vi "Event Status Enable.vi"(0 "Instrument Handle In":i32, 1 "Status Register":i32 format="%02x", 2 "Frequency Register":i32 format="%02x", 3 "Test Register":i32 format="%04x", 4 "Operation Register":i32 format="%04x", 5 "error in":errorcluster, 6 "Standard Register":i32 format="%02x", 7 "Questionable Register":i32 format="%04x", 8 "Voltage Register":i32 format="%02x", 9 "Calibration Register":i32 format="%02x", 10 "Dig1 Register":i32 caption="Digitizer 1 Register" format="%02x", 11 "Dig2 Register":i32 caption="Digitizer 2 Register" format="%02x") -> (14 "Instrument Handle Out":i32, 19 "error out":errorcluster)   [LabVIEW 8.6, in "ZTScopeM.lvlib"]
doc: "Set all error register event forwarding states."
uses:
  ZTScopeM.lvlib
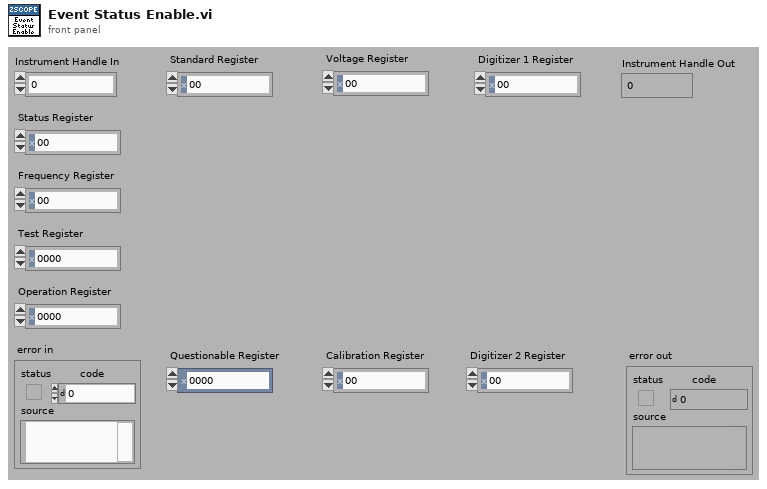
[diagram p1: front panel]
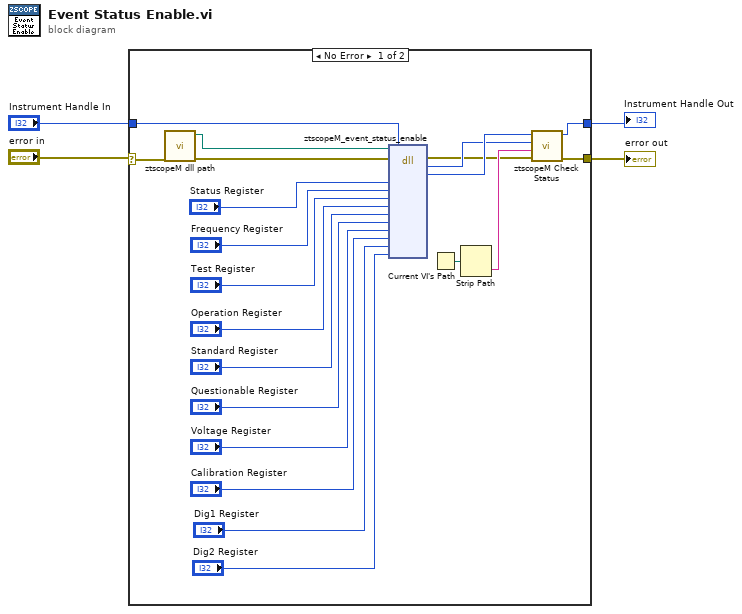
[diagram p0: block diagram]
diagram:
  n1 = case shown="No Error" "error in" {
    selector: "error in" -> [w8 w27]
    tunnel: [w20 w27] -> w1
    tunnel: "Instrument Handle In" -> [w25 w26]
    tunnel: [w19 w26] -> w3
    frame #0 {
      n2 = call "ztscopeM dll path.vi"("error in (no error)"=w8) -> ("error out"=w6:errorcluster, "<instrument>.dll path"=w7:path)  [unwired: 9 in]
      n3 = dll-call lib="C:/Program Files (x86)/National Instruments/LabVIEW 2013/instr.lib/ztscopem/ztscopeM.dll" fn="ztscopeM_event_status_enable"(path in=w7, error in=w6, "instrumentHandle"=w25, "statusRegister"="Status Register", "frequencyRegister"="Frequency Register", "testRegister"="Test Register", "operationRegister"="Operation Register", "standardRegister"="Standard Register", "questionableRegister"="Questionable Register", "voltageRegister"="Voltage Register", "calibrationRegister"="Calibration Register", "dig1Register"="Dig1 Register", "dig2Register"="Dig2 Register") -> (error out=w5:errorcluster, w21:i32, "instrumentHandle"=w22:i32)  [unwired: 11 in, 1 out]
      n4 = Current VI's Path() -> (path=w24:path)
      n5 = Strip Path(path=w24) -> (name=w23:string)  [unwired: 1 out]
      n6 = call "ztscopeM Check Status.vi"("error in"=w5, "name of VI"=w23, "status (return code)"=w21, "instrument handle in"=w22) -> ("error out"=w20:errorcluster, "instrument handle out"=w19:i32)  [unwired: 2 in]
    }
    frame #1 {
    }
  }
  "Instrument Handle Out" <- w3
  "error out" <- w1
